vi "INSPECT_Wait for Inspect Range Helper.vi"(8 "error in (no error)":errorcluster, 10 "Inspect Helper Loop Data":T1={"Inspect State"=enum."Init", "Timeout"=-1, "Loop Count"=0, "Start Sample No."=0, "Inspect Status "={"Ready"=FALSE, "Inspecting"=FALSE, "Cancel"=FALSE}, "Encoder Count"=0, "PosToStartScan"=50800, "ScanLength"=50800, "MaxSamples"=50800, "PosToEndScan"=0, "Host SampleData"=refnum, "data value reference"=refnum, "Block Cnt notifier out"=refnum, "STATUS"={"Initialized"=FALSE, "Connected"=FALSE, "Ready"=FALSE, "Inspecting"=FALSE, "Position"=0.0, "Status"=0, "Error"=FALSE, "Code"=0, "MC SM State"=0, "M_Ctrl"=0}, "EventLog"=refnum}, 11 "Message Queue in":refnum<class "Delacor_lib_QMH_Message Queue.lvclass">) -> (0 "error out":errorcluster, 2 "Inspect Helper Loop Data out":T1={"Inspect State"=enum."Init", "Timeout"=0, "Loop Count"=0, "Start Sample No."=0, "Inspect Status "={"Ready"=FALSE, "Inspecting"=FALSE, "Cancel"=FALSE}, "Encoder Count"=0, "PosToStartScan"=50800, "ScanLength"=50800, "MaxSamples"=50800, "PosToEndScan"=0, "Host SampleData"=refnum, "data value reference"=refnum, "Block Cnt notifier out"=refnum, "STATUS"={"Initialized"=FALSE, "Connected"=FALSE, "Ready"=FALSE, "Inspecting"=FALSE, "Position"=0.0, "Status"=0, "Error"=FALSE, "Code"=0, "MC SM State"=0, "M_Ctrl"=0}, "EventLog"=refnum})   [LabVIEW 2015, in "Tool Module.lvlib"]
uses:
  Tool Module.lvlib
  _Inspect Helper Loop Data Cluster--typedef.ctl
  Event Logger Library/Event Log/EventLog.lvclass
  _Inspect SM Enum--typedef.ctl
  _Inspect Status Update Cluster--typedef.ctl
  _Sample Data Rtn Cluster--typedef.ctl
  _STATUS Typedef--cluster.ctl
  <vilib>/Delacor/Delacor QMH/Libraries/Message Queue_class/Delacor_lib_QMH_Message Queue.lvclass
  _Inspection Limits cluster--typedef.ctl
  <vilib>/Delacor/Delacor QMH/Libraries/Message Queue_class/Delacor_lib_QMH_Message Queue.lvclass/Delacor_lib_QMH_Message Queue.ctl
  <vilib>/Delacor/Delacor QMH/Libraries/Message Queue_class/Delacor_lib_QMH_Enqueue Message (Single).vi
  ToolModGLOB.vi
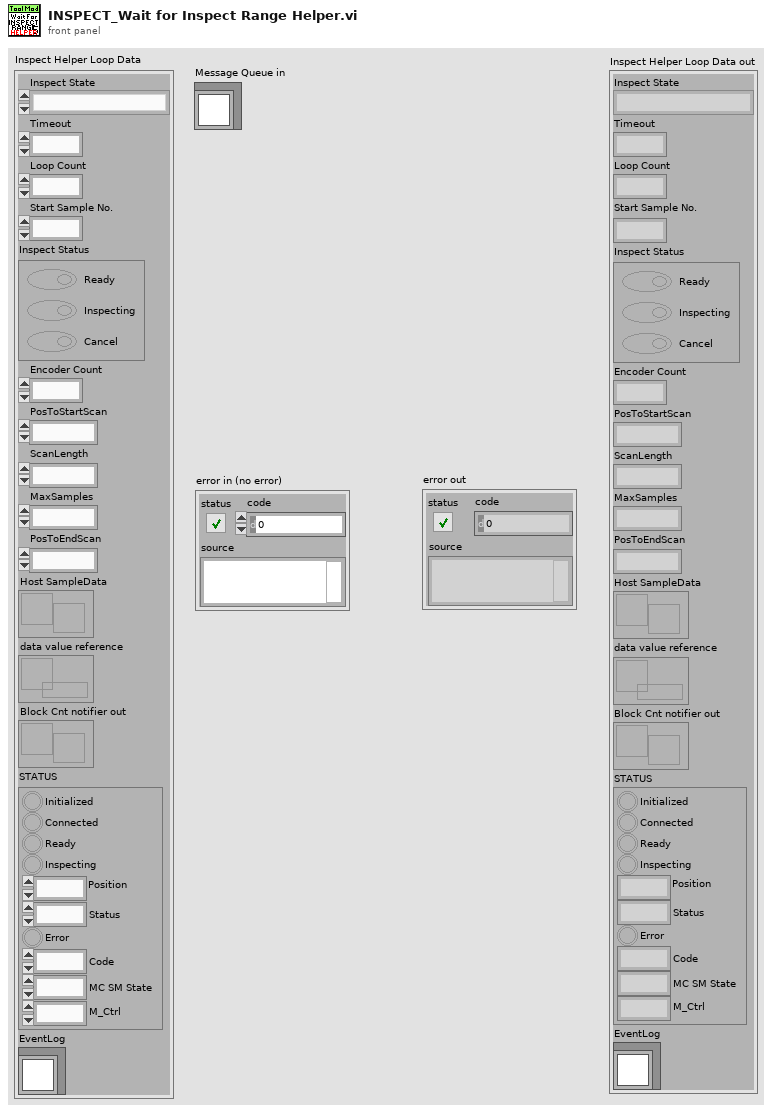
[diagram p1: front panel]
types:
  T1 = typedef "Tool Module.lvlib/_Inspect Helper Loop Data Cluster--typedef.ctl" = cluster{"Inspect State":T2, "Timeout":i32, "Loop Count":i32, "Start Sample No.":u32, "Inspect Status ":T3, "Encoder Count":i32, "PosToStartScan":i32, "ScanLength":i32, "MaxSamples":i32, "PosToEndScan":i32, "Host SampleData":refnum<notifier>, "data value reference":refnum<data-value>, "Block Cnt notifier out":refnum<notifier>, "STATUS":T4, "EventLog":refnum<class "EventLog.lvclass">}
  T2 = typedef "Tool Module.lvlib/_Inspect SM Enum--typedef.ctl" = enum16{"Init", "Set Motion Speed", "Move To Scan Start", "Wait for Motion Out", "Wait for Start Pos", "Delay before Motion IN", "Start Inspecting", "Wait for Motion IN", "Wait for Inspect Range", "Delay before Inspecting", "Inspecting", "Stop Inspecting"}
  T3 = typedef "Tool Module.lvlib/_Inspect Status Update Cluster--typedef.ctl" = cluster{"Ready":bool, "Inspecting":bool, "Cancel":bool}
  T4 = typedef "Tool Module.lvlib/_STATUS Typedef--cluster.ctl" = cluster{"Initialized":bool, "Connected":bool, "Ready":bool, "Inspecting":bool, "Position":dbl, "Status":u16, "Error":bool, "Code":i32, "MC SM State":u16, "M_Ctrl":u16}
  T5 = typedef "Tool Module.lvlib/_Inspection Limits cluster--typedef.ctl" = cluster{"MaxSamples":i32, "PosToStartScan":i32, "PosToEndScan":i32, "ScanLength":i32}
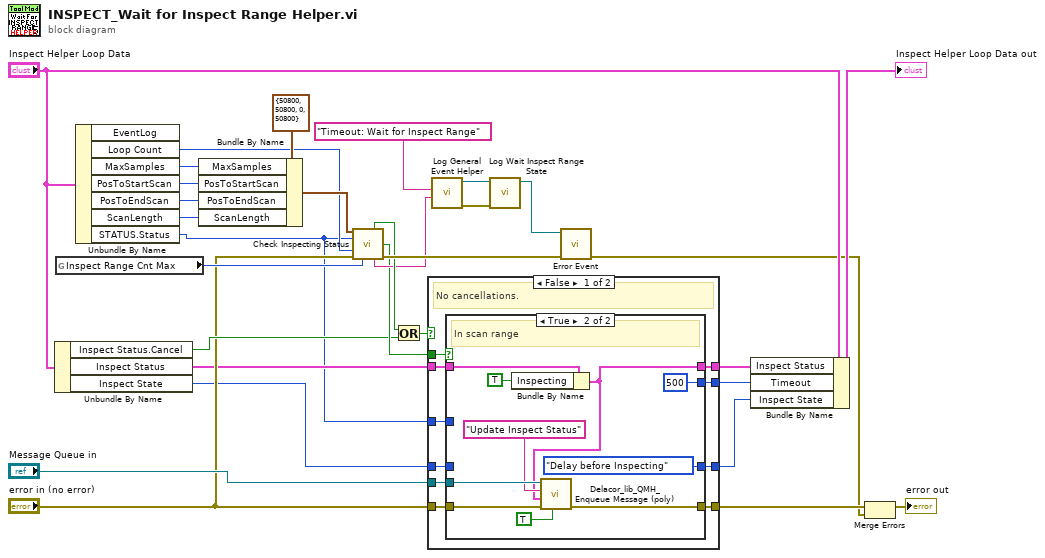
[diagram p0: block diagram]
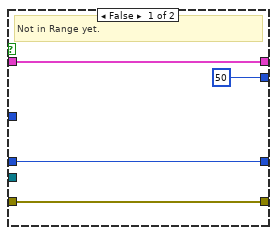
[diagram p2: hidden frame]
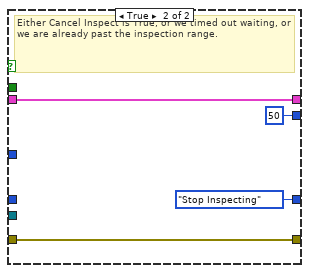
[diagram p3: hidden frame]
diagram:
  n1 = Unbundle By Name("Inspect Helper Loop Data") -> ("Inspect Status.Cancel"=w14:bool, "Inspect Status"=w10:T3, "Inspect State"=w5:T2)
  n2 = global read "ToolModGLOB.vi" "Inspect Range Cnt Max"() -> (w24:i32)
  n3 = Unbundle By Name("Inspect Helper Loop Data") -> ("Loop Count"=w25:i32, "MaxSamples"=w30:i32, "PosToStartScan"=w29:i32, "PosToEndScan"=w28:i32, "ScanLength"=w27:i32, "STATUS.Status"=w6:u16)  [unwired: 1 out]
  n4 = Bundle By Name(cluster=T5 {"MaxSamples"=50800, "PosToStartScan"=50800, "PosToEndScan"=0, "ScanLength"=50800} ("Inspection Limits"), "MaxSamples"=w30, "PosToStartScan"=w29, "PosToEndScan"=w28, "ScanLength"=w27) -> (w26:T5)
  n5 = call "Check Inspecting Status.vi"("Inspection Limits"=w26, "Status Byte"=w6, "Loop Counter"=w25, "error in (no error)"="error in (no error)", "Max Tries"=w24) -> ("Stop Inspection"=w19:bool, "Inside Scan Region"=w15:bool, "DebugLog String"=w18:string, "error out"=w20:errorcluster)  [unwired: 3 in, 4 out]
  n6 = Or(x=w19, y=w14) -> (x .or. y?=w16:bool)
  n7 = case shown="False" w16 {
    tunnel: "error in (no error)" -> [w41 w58]
    tunnel: "Message Queue in" -> [w40 _]
    tunnel: w15 -> [w39 _]
    tunnel: [w38 w58] -> w7
    tunnel: w10 -> [w37 w59]
    tunnel: w6 -> [w36 _]
    tunnel: [w35 w59] -> w11
    tunnel: [w34 _Inspect_SM_Enum--typedef."Stop Inspecting" ("Inspect State")] -> w3
    tunnel: w5 -> [w33 _]
    tunnel: [w32 50 ("Period")] -> w4
    frame False {
      # "No cancellations."
      n8 = case shown="True" w39 {
        tunnel: w41 -> [w42 w52]
        tunnel: w40 -> [_ w53]
        tunnel: [w42 w48] -> w38
        tunnel: w37 -> [w45 w55]
        tunnel: w36 -> [_ _]
        tunnel: [w45 w49] -> w35
        tunnel: [w43 _Inspect_SM_Enum--typedef."Delay before Inspecting" ("Inspect State")] -> w34
        tunnel: w33 -> [w43 _]
        tunnel: [50 ("Period") 500 ("Period")] -> w32
        frame False {
          # "Not in Range yet."
        }
        frame True {
          # "In scan range"
          n9 = Bundle By Name(cluster=w55, "Inspecting"=TRUE) -> (w49:T3)
          n10 = call-poly <vilib>:"Delacor_lib_QMH_Enqueue Message (poly).vi"("Priority Message? (F)"=TRUE, "error in (no error)"=w52, "Message Data"=w49, "Message"="Update Inspect Status", "Message Queue in"=w53) -> ("error out"=w48:errorcluster)  [unwired: 5 in, 1 out]
        }
      }
    }
    frame True {
      # "Either Cancel Inspect is True, or we timed out waiting, or we are already past the inspection range."
    }
  }
  n11 = call "Log General Event Helper.vi"("Payload"=w18, "State Info"="Timeout: Wait for Inspect Range") -> ("error out"=w22:errorcluster, "EventLog out"=w21:refnum<class "EventLog.lvclass">)  [unwired: 8 in]
  n12 = call "Log Wait Inspect Range State.vi"("error in (no error)"=w22, "EventLog in"=w21) -> ("EventLog out"=w23:refnum<class "EventLog.lvclass">)  [unwired: 8 in, 1 out]
  n13 = call "Error Event.vi"("error in (no error)"=w20, "EventLog ref"=w23) -> ("error out"=w1:errorcluster)  [unwired: 8 in, 1 out]
  n14 = Bundle By Name(cluster="Inspect Helper Loop Data", "Inspect Status"=w11, "Timeout"=w4, "Inspect State"=w3) -> (→"Inspect Helper Loop Data out":T1)
  n15 = Merge Errors(w7, w1) -> (→"error out":errorcluster)
